vi "ProdaNG.Convert.DBL-U8[].vi"(11 "dbl":dbl) -> (3 "unsigned byte array":u8[](array[numeric]))   [LabVIEW 2016]
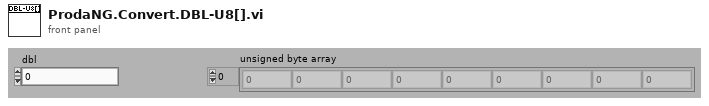
[diagram p1: front panel]
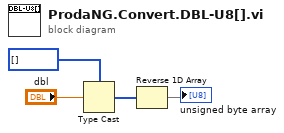
[diagram p0: block diagram]
diagram:
  n1 = Type Cast(type=u8[] [] ("unsigned byte array"), x="dbl") -> (*(type *) &x=w4:u8[])
  n2 = Reverse 1D Array(array=w4) -> (reversed array=→"unsigned byte array":u8[])
